vi "溶解氧 随机数出数.vi"(9 "原始值":dbl) -> (2 "信号值":dbl, 3 "取值输出":dbl, 4 "x .and. y?":bool)   [LabVIEW 2016]
uses:
  Holding Var.vi
  Process var.vi
  random number/random number.lvlib
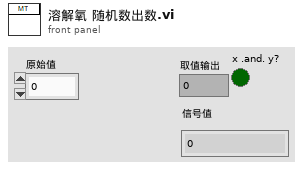
[diagram p1: front panel]
types:
  T1 = cluster{"水温":cluster{"参数输入":cluster{"采样模式":enum16{"自动采样", "手动采样"}, "采样点数":i32, "变异系数设定值":dbl, "重新取值百分比":dbl, "偏差模式":enum16{"相对偏差", "绝对偏差"}, "相对偏差百分比":dbl, "绝对偏差值":dbl}, "采样值":dbl[], "启用":bool}, "pH":cluster{"参数输入":cluster{"采样模式":enum16{"自动采样", "手动采样"}, "采样点数":i32, "变异系数设定值":dbl, "重新取值百分比":dbl, "偏差模式":enum16{"相对偏差", "绝对偏差"}, "相对偏差百分比":dbl, "绝对偏差值":dbl}, "采样值":dbl[], "启用":bool}, "DO%":cluster{"参数输入":cluster{"采样模式":enum16{"自动采样", "手动采样"}, "采样点数":i32, "变异系数设定值":dbl, "重新取值百分比":dbl, "偏差模式":enum16{"相对偏差", "绝对偏差"}, "相对偏差百分比":dbl, "绝对偏差值":dbl}, "采样值":dbl[], "启用":bool}, "电导率":cluster{"参数输入":cluster{"采样模式":enum16{"自动采样", "手动采样"}, "采样点数":i32, "变异系数设定值":dbl, "重新取值百分比":dbl, "偏差模式":enum16{"相对偏差", "绝对偏差"}, "相对偏差百分比":dbl, "绝对偏差值":dbl}, "采样值":dbl[], "启用":bool}, "浊度":cluster{"参数输入":cluster{"采样模式":enum16{"自动采样", "手动采样"}, "采样点数":i32, "变异系数设定值":dbl, "重新取值百分比":dbl, "偏差模式":enum16{"相对偏差", "绝对偏差"}, "相对偏差百分比":dbl, "绝对偏差值":dbl}, "采样值":dbl[], "启用":bool}}
  T2 = cluster{"采样模式":enum16{"自动采样", "手动采样"}, "采样点数":i32, "变异系数设定值":dbl, "重新取值百分比":dbl, "偏差模式":enum16{"相对偏差", "绝对偏差"}, "相对偏差百分比":dbl, "绝对偏差值":dbl}
  T3 = cluster{"水温":cluster{"mean":dbl, "变异系数":dbl, "随机数？":bool}, "pH":cluster{"mean":dbl, "变异系数":dbl, "随机数？":bool}, "DO":cluster{"mean":dbl, "变异系数":dbl, "随机数？":bool}, "电导率":cluster{"mean":dbl, "变异系数":dbl, "随机数？":bool}, "浊度":cluster{"mean":dbl, "变异系数":dbl, "随机数？":bool}}
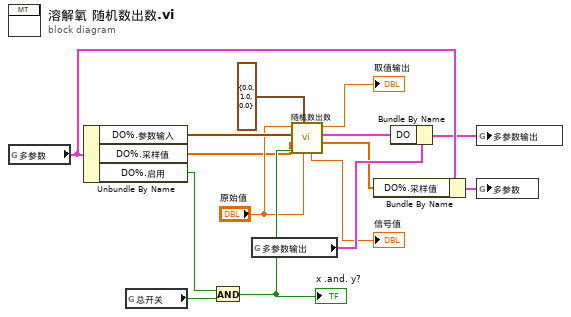
[diagram p0: block diagram]
diagram:
  n1 = global read "Holding Var.vi" "多参数"() -> (w15:T1)
  n2 = Unbundle By Name(w15) -> ("DO%.参数输入"=w8:T2, "DO%.采样值"=w1:dbl[], "DO%.启用"=w6:bool)
  n3 = global read "Holding Var.vi" "总开关"() -> (w11:bool)
  n4 = And(x=w6, y=w11) -> (x .and. y?=w5:bool)
  "x .and. y?" <- w5
  n5 = global read "Process var.vi" "多参数输出"() -> (w14:T3)
  n6 = call "随机数出数.vi"("信号值原始值"="原始值", "公式"=cluster{"X^2":dbl, "X":dbl, "B":dbl} {"X^2"=0.0, "X"=1.0, "B"=0.0}, "启用"=w5, "采样值"=w1, "参数输入"=w8, "监测值原始值"="原始值") -> ("采样值输出"=w4:dbl[], "参数输出"=w7:cluster{"mean":dbl, "变异系数":dbl, "随机数？":bool}, "取值输出"=→"取值输出":dbl, "信号值"=→"信号值":dbl)  [unwired: 2 in]
  n7 = Bundle By Name(cluster=w15, "DO%.采样值"=w4) -> (w9:T1)
  n8 = Bundle By Name(cluster=w14, "DO"=w7) -> (w13:T3)
  n9 = global write "Process var.vi" "多参数输出"(w13) -> ()
  n10 = global write "Holding Var.vi" "多参数"(w9) -> ()
